vi "unbundle mappings by action channel classification.vi"(10 "channel":refnum<class "TBM channel.lvclass">, 11 "Mappings":T4) -> (1 "Mappings For One Method":T1[](array[typedef]), 2 "channel out":refnum<class "TBM channel.lvclass">, 3 "Mappings out":T4)   [LabVIEW 2014, in "base TBM sequencer configuration.lvclass"]
uses:
  base TBM sequencer configuration.lvclass
  Module Mappings.ctl
  <vilib>/NI/Tag Bus/table/mapping specification.ctl
  <vilib>/NI/Tag Bus/tag/Data Type.ctl
  <vilib>/NI/Tag Bus/table/mapping.ctl
  <vilib>/NI/Tag Bus Module Framework/channel/TBM channel.lvclass
  <vilib>/NI/Tag Bus Module Framework/channel/TBM channel.lvclass/TBM channel.ctl
  <vilib>/NI/Tag Bus Module Framework/channel/Read channel classification.vi
  <vilib>/NI/Tag Bus/tag/tag descriptor.lvclass
  <vilib>/NI/Tag Bus/table/data table.lvlib
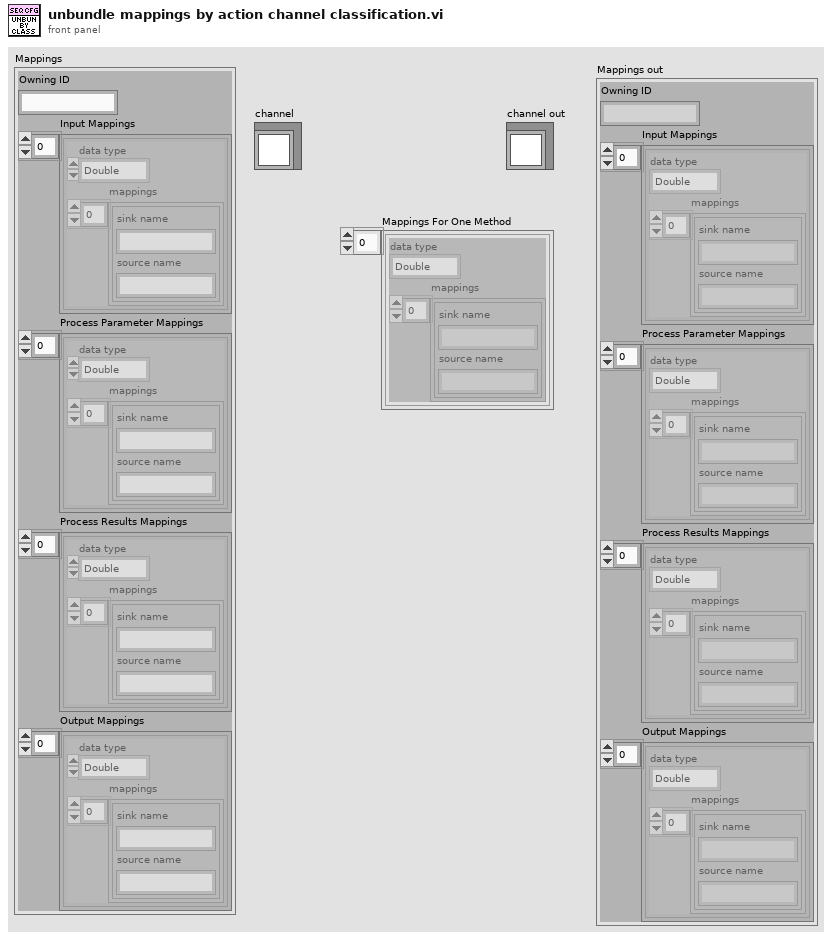
[diagram p1: front panel]
types:
  T1 = typedef "tag bus.lvlib/data table.lvlib/mapping specification.ctl" = cluster{"data type":T2, "mappings":T3[]}
  T2 = typedef "tag bus.lvlib/tag descriptor.lvclass/Data Type.ctl" = enum16{"Double", "Single", "I64", "I32", "I16", "I8", "U64", "U32", "U16", "U8", "Boolean", "String", "Array of Double", "Array of Single", "Array of I64", "Array of I32", "Array of I16", "Array of I8", "Array of U64", "Array of U32", "Array of U16", "Array of U8", "Array of Boolean", "Array of String"}
  T3 = typedef "tag bus.lvlib/data table.lvlib/mapping.ctl" = cluster{"sink name":string, "source name":string}
  T4 = typedef "base TBM sequencer configuration.lvclass/Module Mappings.ctl" = cluster{"Owning ID":string, "Input Mappings":T1[], "Process Parameter Mappings":T1[], "Process Results Mappings":T1[], "Output Mappings":T1[]}
  T5 = typedef "TBM channel.lvclass/channel classification.ctl" = enum16{"input data", "output data", "processing parameter", "processing result"}
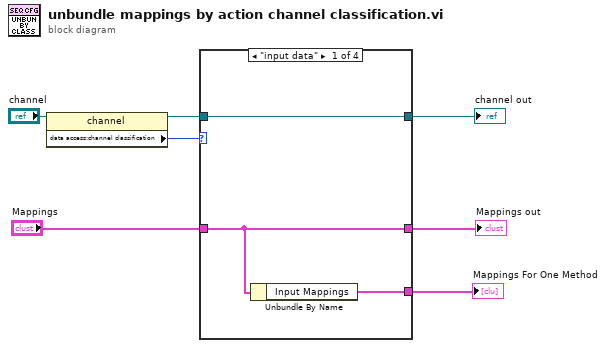
[diagram p0: block diagram]
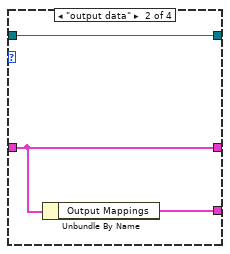
[diagram p2: hidden frame]
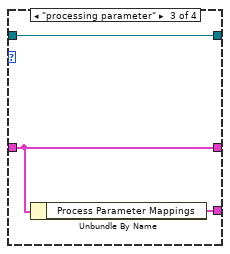
[diagram p3: hidden frame]
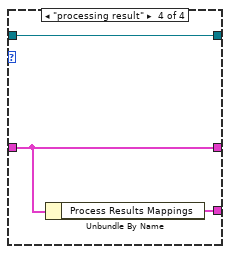
[diagram p4: hidden frame]
diagram:
  n1 = property class="channel"(reference="channel") -> (reference out=w5:refnum<class "TBM channel.lvclass">, "data access:channel classification"=w6:T5)  [unwired: 1 in, 1 out]
  n2 = case shown="\"input data\"" w6 {
    tunnel: "Mappings" -> [w9 w12 w14 w17]
    tunnel: [w9 w12 w14 w17] -> w2
    tunnel: [w10 w13 w16 w18] -> w1
    tunnel: w5 -> [w8 w11 w15 w19]
    tunnel: [w8 w11 w15 w19] -> w4
    frame "input data" {
      n3 = Unbundle By Name(w9) -> ("Input Mappings"=w10:T1[])
    }
    frame "output data" {
      n4 = Unbundle By Name(w12) -> ("Output Mappings"=w13:T1[])
    }
    frame "processing parameter" {
      n5 = Unbundle By Name(w14) -> ("Process Parameter Mappings"=w16:T1[])
    }
    frame "processing result" {
      n6 = Unbundle By Name(w17) -> ("Process Results Mappings"=w18:T1[])
    }
  }
  "Mappings out" <- w2
  "channel out" <- w4
  "Mappings For One Method" <- w1
